vi "logScanSettings.vi"(8 "error in (no error)":errorcluster, 11 "Model in":refnum<class "Model.lvclass">) -> (0 "error out":errorcluster, 3 "Model out":refnum<class "Model.lvclass">)   [LabVIEW 2015, in "Model.lvclass"]
uses:
  Model.lvclass
  Model.lvclass/Model.ctl
  TestLog/ITestLog/ITestLog.lvclass
  Actuator/IActuator/IActuator.lvclass
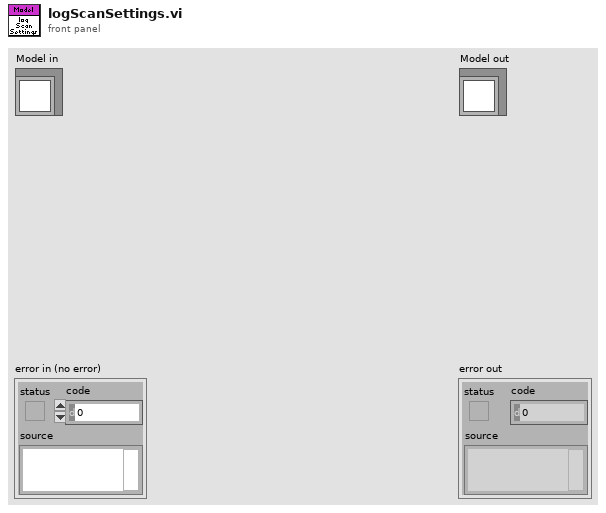
[diagram p1: front panel]
types:
  T1 = typedef "FAMTTypedefs.lvlib/Waveform.ctl" = enum16{"Sine", "Triangle", "Square", "Sawtooth", "Chirp", "Gaussian", "Trapezoid"}
  T2 = typedef "FAMTTypedefs.lvlib/Flow Control Settings.ctl" = cluster{"DAC Channel":u8, "ROT Bias":u8, "Minimum Voltage":dbl, "Maximum Voltage":dbl, "Off Value":dbl, "Closed Loop Settings":T3}
  T3 = typedef "FAMTTypedefs.lvlib/ClosedLoopSettings.ctl" = cluster{"P":dbl, "I":dbl, "D":dbl, "Minimum":dbl, "Maximum":dbl}
  T4 = typedef "FAMTTypedefs.lvlib/Pressure Servo Settings.ctl" = cluster{"Center Point":dbl[unit], "Area":dbl, "PA to PSI":dbl, "Servo 1 DAC Channel":u8, "Servo 2 DAC Channel":u8, "Closed Loop Settings":T3, "Off Value":dbl}
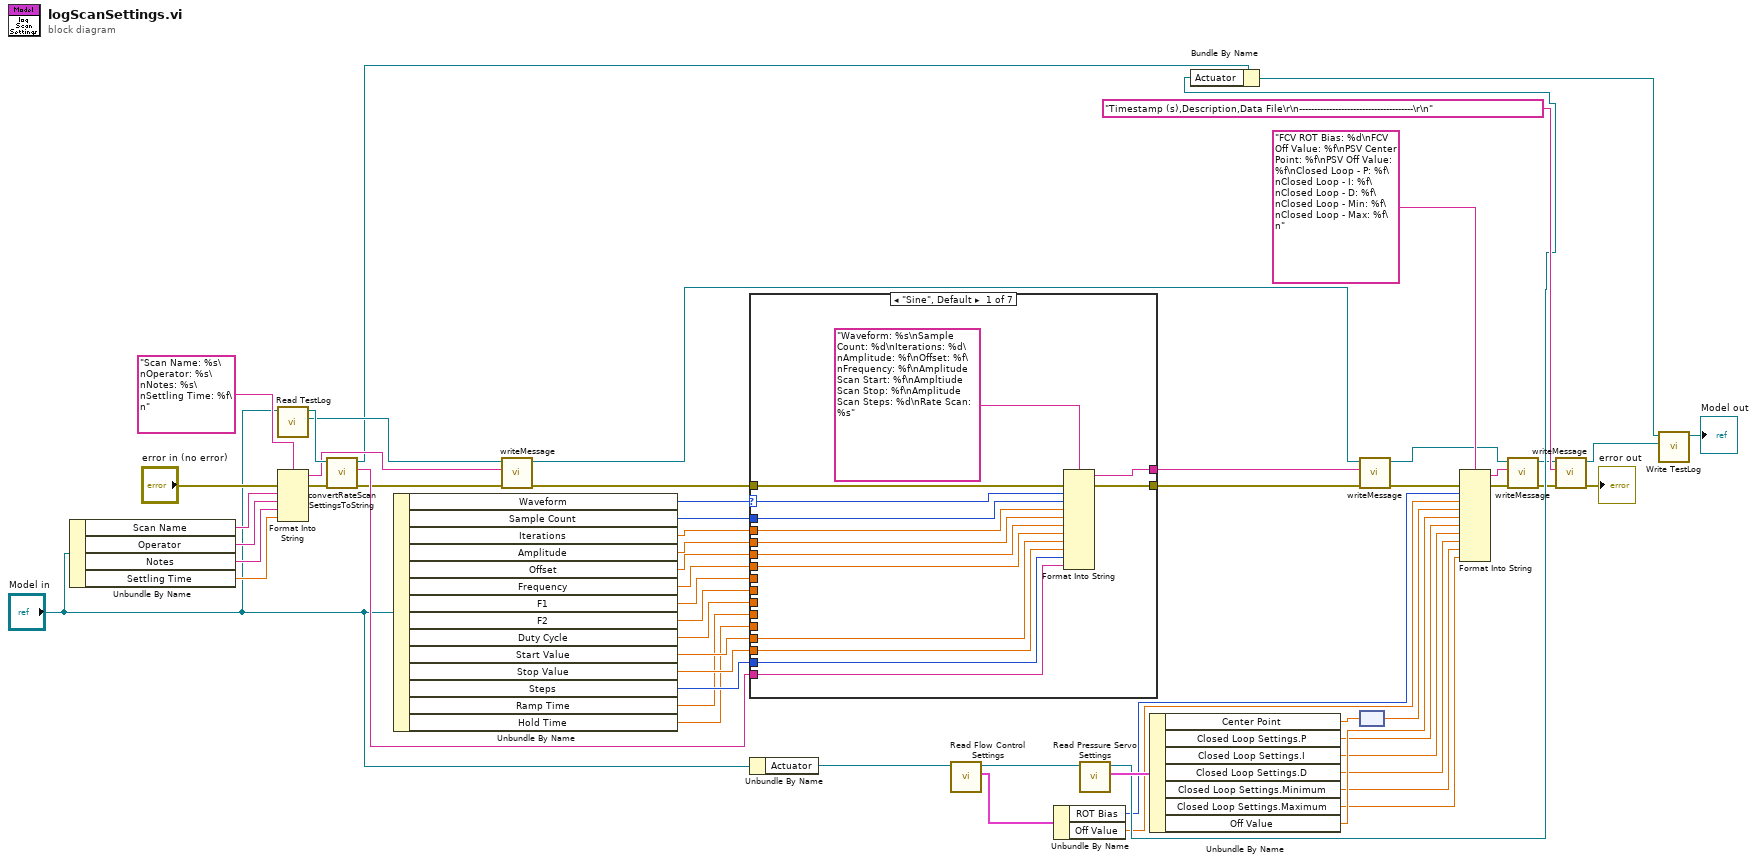
[diagram p0: block diagram]
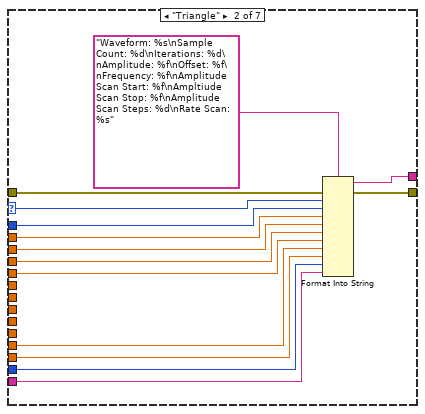
[diagram p2: hidden frame]
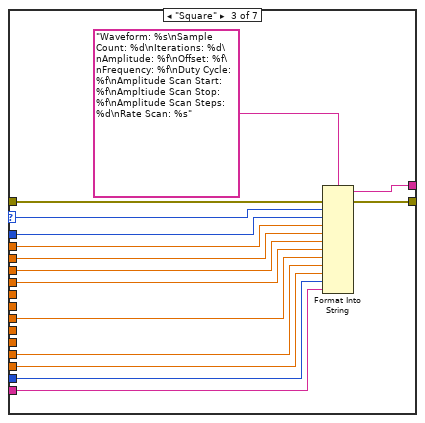
[diagram p3: hidden frame]
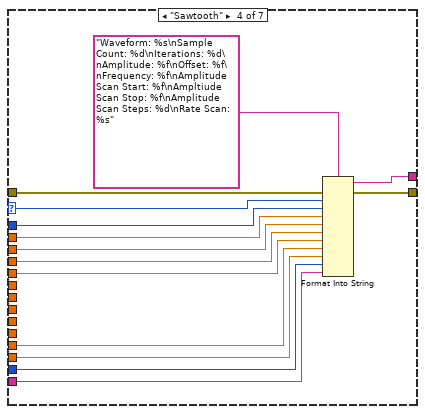
[diagram p4: hidden frame]
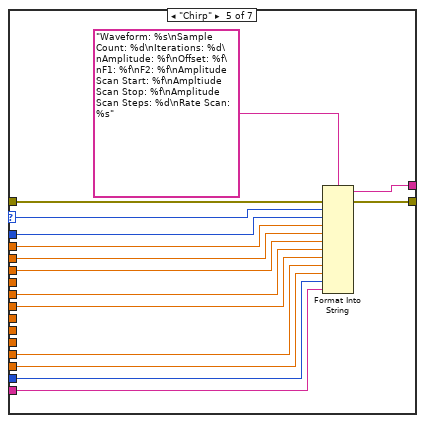
[diagram p5: hidden frame]
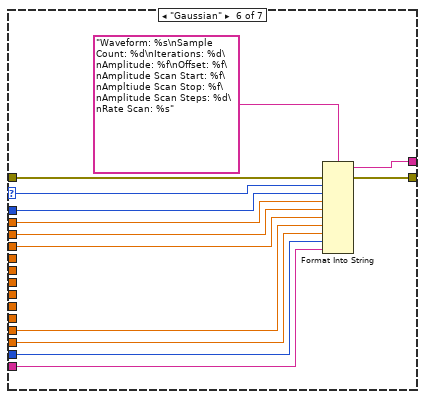
[diagram p6: hidden frame]
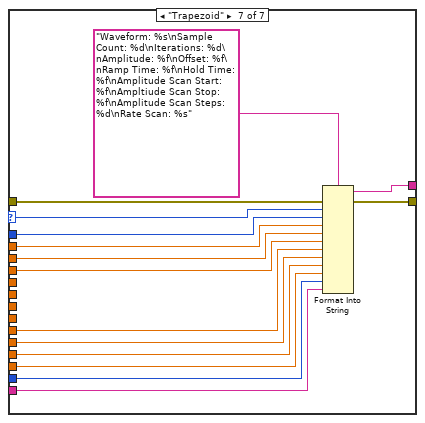
[diagram p7: hidden frame]
diagram:
  n1 = Unbundle By Name("Model in") -> ("Scan Name"=w42:string, "Operator"=w41:string, "Notes"=w40:string, "Settling Time"=w26:dbl[unit])
  n2 = call "Read TestLog.vi"("Model in"="Model in") -> ("ITestLog.lvclass"=w39:refnum<class "ITestLog.lvclass">, "Model out"=w59:refnum<class "Model.lvclass">)  [unwired: 9 in]
  n3 = Format Into String(format string="Scan Name: %s\nOperator: %s\nNotes: %s\nSettling Time: %f\n", error in="error in (no error)", w42, w41, w40, w26) -> (resulting string=w37:string, error out=w33:errorcluster)  [unwired: 1 in]
  n4 = call "convertRateScanSettingsToString.vi"("error in (no error)"=w33, "Model in"=w59) -> ("error out"=w32:errorcluster, "Rate Scan Settings"=w46:string, "Model out"=w19:refnum<class "Model.lvclass">)  [unwired: 7 in]
  n5 = Unbundle By Name("Model in") -> ("Waveform"=w58:T1, "Sample Count"=w57:u32, "Iterations"=w56:dbl, "Amplitude"=w55:dbl, "Offset"=w54:dbl, "Frequency"=w53:dbl[unit], "F1"=w52:dbl[unit], "F2"=w51:dbl[unit], "Duty Cycle"=w50:dbl, "Start Value"=w49:dbl, "Stop Value"=w48:dbl, "Steps"=w47:u16, "Ramp Time"=w28:dbl[unit], "Hold Time"=w27:dbl[unit])
  n6 = call-dynamic "writeMessage.vi"("error in (no error)"=w32, "Message"=w37, "ITestLog in"=w39) -> ("error out"=w31:errorcluster, "ITestLog out"=w38:refnum<class "ITestLog.lvclass">)  [unwired: 7 in]
  n7 = case shown="\"Sine\", Default" w58 {
    selector: w58 -> [w72 w82 w97 w115 w129 w143 w158]
    tunnel: w57 -> [w71 w81 w96 w114 w128 w142 w157]
    tunnel: w56 -> [w70 w80 w95 w113 w127 w141 w156]
    tunnel: w55 -> [w69 w79 w94 w112 w126 w140 w155]
    tunnel: w54 -> [w68 w78 w93 w111 w125 w139 w154]
    tunnel: w53 -> [w67 w83 w92 w110 _ _ _]
    tunnel: w52 -> [_ _ _ _ w124 _ _]
    tunnel: w51 -> [_ _ _ _ w123 _ _]
    tunnel: w50 -> [_ _ w91 _ _ _ _]
    tunnel: w49 -> [w66 w84 w98 w109 w122 w138 w153]
    tunnel: w48 -> [w65 w85 w99 w108 w121 w137 w152]
    tunnel: w47 -> [w64 w86 w100 w107 w120 w136 w151]
    tunnel: w46 -> [w63 w77 w101 w106 w130 w135 w150]
    tunnel: [w62 w76 w90 w105 w119 w134 w149] -> w45
    tunnel: w31 -> [w61 w75 w89 w104 w118 w133 w148]
    tunnel: [w60 w74 w88 w103 w117 w132 w147] -> w30
    tunnel: w28 -> [_ _ _ _ _ _ w146]
    tunnel: w27 -> [_ _ _ _ _ _ w145]
    frame "Sine", Default {
      n8 = Format Into String(format string="Waveform: %s\nSample Count: %d\nIterations: %d\nAmplitude: %f\nOffset: %f\nFrequency: %f\nAmplitude Scan Start: %f\nAmpltiude Scan Stop: %f\nAmplitude Scan Steps: %d\nRate Scan: %s", error in=w61, w72, w71, w70, w69, w68, w67, w66, w65, w64, w63) -> (resulting string=w62:string, error out=w60:errorcluster)  [unwired: 1 in]
    }
    frame "Triangle" {
      n9 = Format Into String(format string="Waveform: %s\nSample Count: %d\nIterations: %d\nAmplitude: %f\nOffset: %f\nFrequency: %f\nAmplitude Scan Start: %f\nAmpltiude Scan Stop: %f\nAmplitude Scan Steps: %d\nRate Scan: %s", error in=w75, w82, w81, w80, w79, w78, w83, w84, w85, w86, w77) -> (resulting string=w76:string, error out=w74:errorcluster)  [unwired: 1 in]
    }
    frame "Square" {
      n10 = Format Into String(format string="Waveform: %s\nSample Count: %d\nIterations: %d\nAmplitude: %f\nOffset: %f\nFrequency: %f\nDuty Cycle: %f\nAmplitude Scan Start: %f\nAmpltiude Scan Stop: %f\nAmplitude Scan Steps: %d\nRate Scan: %s", error in=w89, w97, w96, w95, w94, w93, w92, w91, w98, w99, w100, w101) -> (resulting string=w90:string, error out=w88:errorcluster)  [unwired: 1 in]
    }
    frame "Sawtooth" {
      n11 = Format Into String(format string="Waveform: %s\nSample Count: %d\nIterations: %d\nAmplitude: %f\nOffset: %f\nFrequency: %f\nAmplitude Scan Start: %f\nAmpltiude Scan Stop: %f\nAmplitude Scan Steps: %d\nRate Scan: %s", error in=w104, w115, w114, w113, w112, w111, w110, w109, w108, w107, w106) -> (resulting string=w105:string, error out=w103:errorcluster)  [unwired: 1 in]
    }
    frame "Chirp" {
      n12 = Format Into String(format string="Waveform: %s\nSample Count: %d\nIterations: %d\nAmplitude: %f\nOffset: %f\nF1: %f\nF2: %f\nAmplitude Scan Start: %f\nAmpltiude Scan Stop: %f\nAmplitude Scan Steps: %d\nRate Scan: %s", error in=w118, w129, w128, w127, w126, w125, w124, w123, w122, w121, w120, w130) -> (resulting string=w119:string, error out=w117:errorcluster)  [unwired: 1 in]
    }
    frame "Gaussian" {
      n13 = Format Into String(format string="Waveform: %s\nSample Count: %d\nIterations: %d\nAmplitude: %f\nOffset: %f\nAmplitude Scan Start: %f\nAmpltiude Scan Stop: %f\nAmplitude Scan Steps: %d\nRate Scan: %s", error in=w133, w143, w142, w141, w140, w139, w138, w137, w136, w135) -> (resulting string=w134:string, error out=w132:errorcluster)  [unwired: 1 in]
    }
    frame "Trapezoid" {
      n14 = Format Into String(format string="Waveform: %s\nSample Count: %d\nIterations: %d\nAmplitude: %f\nOffset: %f\nRamp Time: %f\nHold Time: %f\nAmplitude Scan Start: %f\nAmpltiude Scan Stop: %f\nAmplitude Scan Steps: %d\nRate Scan: %s", error in=w148, w158, w157, w156, w155, w154, w146, w145, w153, w152, w151, w150) -> (resulting string=w149:string, error out=w147:errorcluster)  [unwired: 1 in]
    }
  }
  n15 = Unbundle By Name("Model in") -> ("Actuator"=w23:refnum<class "IActuator.lvclass">)
  n16 = call-dynamic "Read Flow Control Settings.vi"("IActuator in"=w23) -> ("Flow Control Settings"=w22:T2, "IActuator out"=w24:refnum<class "IActuator.lvclass">)  [unwired: 9 in]
  n17 = Unbundle By Name(w22) -> ("ROT Bias"=w16:u8, "Off Value"=w15:dbl)
  n18 = call-dynamic "Read Pressure Servo Settings.vi"("IActuator in"=w24) -> ("Pressure Servo Settings"=w21:T4, "IActuator out"=w20:refnum<class "IActuator.lvclass">)  [unwired: 9 in]
  n19 = Unbundle By Name(w21) -> ("Center Point"=w2:dbl[unit], "Closed Loop Settings.P"=w13:dbl, "Closed Loop Settings.I"=w12:dbl, "Closed Loop Settings.D"=w11:dbl, "Closed Loop Settings.Minimum"=w10:dbl, "Closed Loop Settings.Maximum"=w9:dbl, "Off Value"=w14:dbl)
  n20 = Bundle By Name(cluster=w19, "Actuator"=w20) -> (w18:refnum<class "Model.lvclass">)
  n21 = call-dynamic "writeMessage.vi"("error in (no error)"=w30, "Message"=w45, "ITestLog in"=w38) -> ("error out"=w8:errorcluster, "ITestLog out"=w4:refnum<class "ITestLog.lvclass">)  [unwired: 7 in]
  n22 = node(w2) -> (w1:dbl)
  n23 = Format Into String(format string="FCV ROT Bias: %d\nFCV Off Value: %f\nPSV Center Point: %f\nPSV Off Value: %f\nClosed Loop - P: %f\nClosed Loop - I: %f\nClosed Loop - D: %f\nClosed Loop - Min: %f\nClosed Loop - Max: %f\n", error in=w8, w16, w15, w1, w14, w13, w12, w11, w10, w9) -> (resulting string=w5:string, error out=w7:errorcluster)  [unwired: 1 in]
  n24 = call-dynamic "writeMessage.vi"("error in (no error)"=w7, "Message"=w5, "ITestLog in"=w4) -> ("error out"=w6:errorcluster, "ITestLog out"=w3:refnum<class "ITestLog.lvclass">)  [unwired: 7 in]
  n25 = call-dynamic "writeMessage.vi"("error in (no error)"=w6, "Message"="Timestamp (s),Description,Data File\r\n--------------------------------------\r\n", "ITestLog in"=w3) -> ("error out"=→"error out":errorcluster, "ITestLog out"=w35:refnum<class "ITestLog.lvclass">)  [unwired: 7 in]
  n26 = call "Write TestLog.vi"("ITestLog.lvclass"=w35, "Model in"=w18) -> ("Model out"=→"Model out":refnum<class "Model.lvclass">)  [unwired: 9 in]
